vi "ASK Receiver.vi"() -> ()   [LabVIEW 2015]
uses:
  <vilib>/addons/Modulation/Analog/support/mod_Set Error Source.vi
  <vilib>/addons/Modulation/Digital/General/MT Generate ASK system parameters (M).vi
  <vilib>/addons/Modulation/Digital/Support/Common/Validators/mod_Generate Filter Coefficients Validate.vi
  <vilib>/addons/Modulation/Digital/General/subVIs/mod_Generate Filter Coefficients.vi
  <instrlib>/niUSRP/niUSRP Fetch Rx Data (CDB Cluster).vi
  <vilib>/addons/Modulation/niDMT.lvlib
panel:
  out "Waveform Graph":cluster{"t0":dbl, "dt":dbl, "Y":dbl[]}[](graph)
  out "XY Graph":T1(graph)
  out "output bit stream":i8[](array[numeric])
  out "Waveform Graph 2":i8[](graph)
  in  "synchronization parameters":T2 {"sync sequence" format="%.2f"}
  in  "pulse shaping filter (none)":T3(ring)
  in  "M-ASK (2)":i32=2
  in  "active antenna":string
  in  "number of samples":i64=1000
  out "coerced gain":dbl format="%#_6f"
  out "coerced carrier frequency":dbl=100000.0 format="%#_6p"
  out "coerced IQ rate":dbl=100000.0 format="%#_6p"
  in  "gain":dbl format="%#_6f"
  in  "carrier frequency":dbl=100000.0 format="%#_6p"
  in  "IQ rate":dbl=100000.0 format="%#_6p"
  in  "y":bool
  in  "device names":refnum<k15>
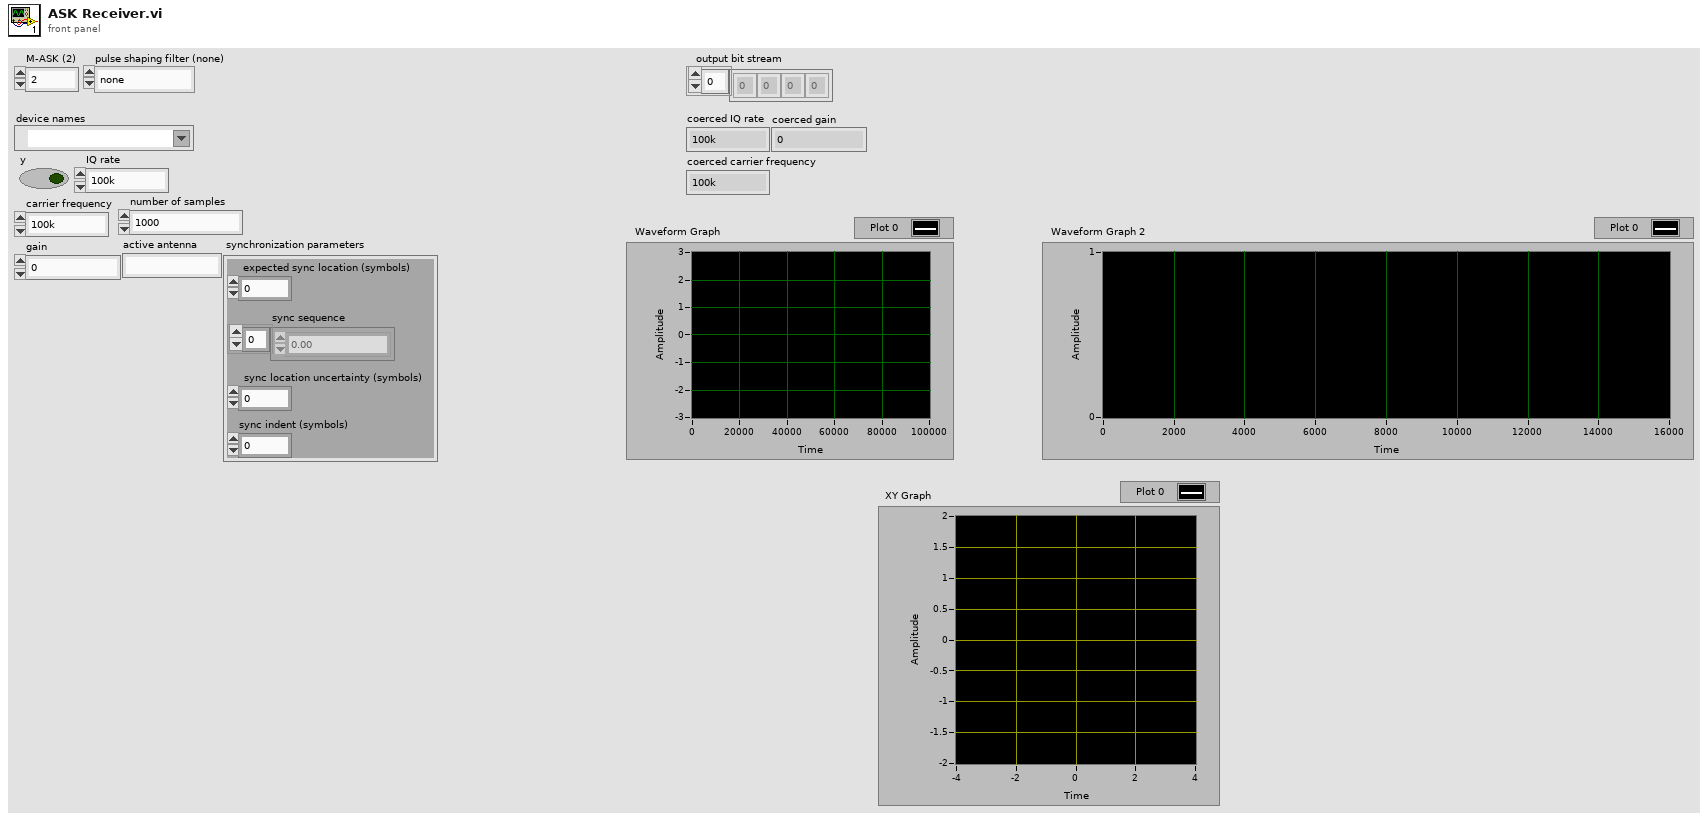
[diagram p1: front panel]
types:
  T1 = cluster{"constellation":dbl[], "oversampled data":dbl[]}[]
  T2 = cluster{"expected sync location (symbols)":i32, "sync sequence":cdb[], "sync location uncertainty (symbols)":i32, "sync indent (symbols)":i32}
  T3 = enum16{"none", "Raised Cosine", "Root Raised Cos", "Gaussian"}
  T4 = enum16{"FSK", "PSK", "QAM", "MSK", "PAM", "ASK", "CPM"}
  T5 = cluster{"samples per symbol (16)":i32, "symbol map":cdb[]}
  T6 = typedef "niAMT.lvlib/Complex Data Waveform.ctl" = cluster{"t0":dbl, "dt":dbl, "Y":cdb[]}
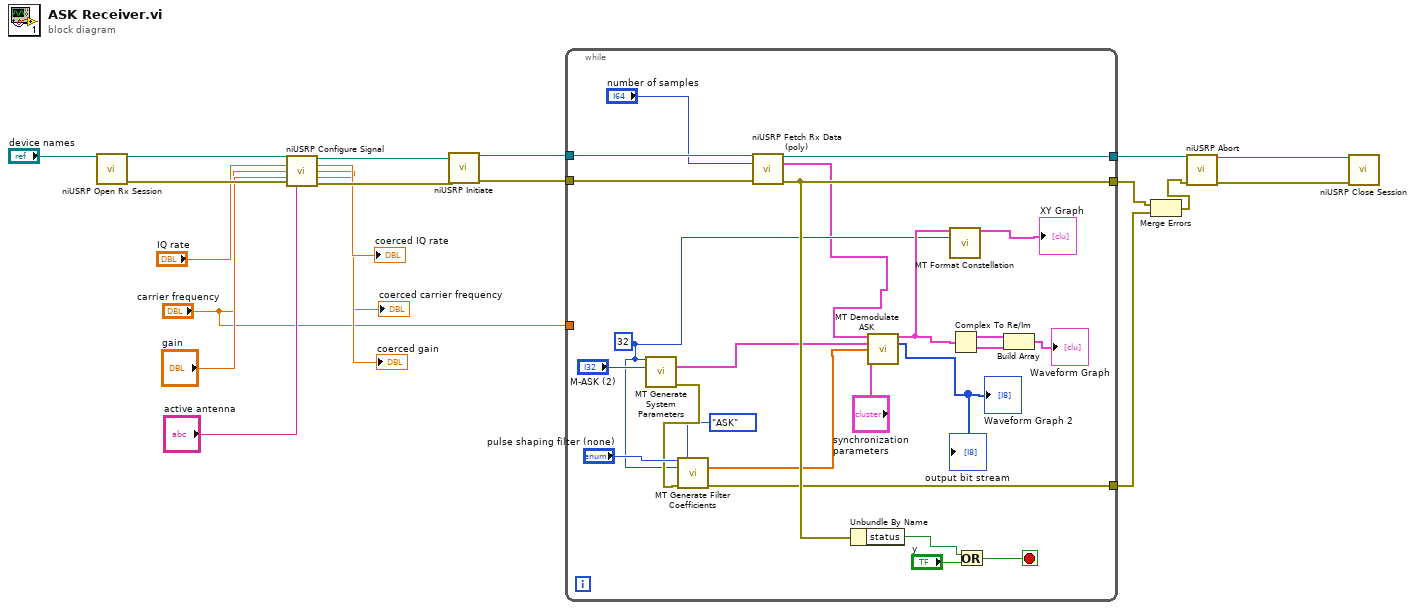
[diagram p0: block diagram]
diagram:
  n1 = call <instrlib>:"niUSRP Open Rx Session.vi"("device names"="device names") -> ("session handle out"=w19:refnum<k15>, "error out"=w17:errorcluster)  [unwired: 13 in]
  n2 = call <instrlib>:"niUSRP Configure Signal.vi"("session handle"=w19, "IQ rate"="IQ rate", "carrier frequency"="carrier frequency", "gain"="gain", "error in (no error)"=w17, "active antenna"="active antenna") -> ("session handle out"=w18:refnum<k15>, "coerced IQ rate"=→"coerced IQ rate":dbl, "coerced carrier frequency"=→"coerced carrier frequency":dbl, "coerced gain"=→"coerced gain":dbl, "error out"=w16:errorcluster)  [unwired: 5 in]
  n3 = call <instrlib>:"niUSRP Initiate.vi"("session handle"=w18, "error in (no error)"=w16) -> ("session handle out"=w15:refnum<k15>, "error out"=w12:errorcluster)  [unwired: 12 in]
  n4 = while {
    tunnel: w15 -> [w44]
    tunnel: [w43] -> w14
    tunnel: w12 -> [w42]
    tunnel: [w38] -> w3
    tunnel: "carrier frequency" -> [_]
    tunnel: [w29] -> w2
    stop <- w41 stop-if-true
    w23 = 32 ("samples per symbol (16)")
    n5 = call-poly <vilib>:"MT Generate System Parameters.vi"("samples per symbol (16)"=w23, "M-ASK (2)"="M-ASK (2)") -> ("ASK system parameters"=w34:T5, "error out"=w30:errorcluster)  [unwired: 11 in, 1 out]
    n6 = call <vilib>:"MT Generate Filter Coefficients.vi"("pulse shaping filter (none)"="pulse shaping filter (none)", "modulation type"=T4."ASK", "pulse shaping samples per symbol (16)"=w23, "error in (no error)"=w30) -> ("matched filter coefficients"=w32:dbl[], "error out"=w29:errorcluster)  [unwired: 9 in, 1 out]
    n7 = call-poly <instrlib>:"niUSRP Fetch Rx Data (poly).vi"("session handle"=w44, "number of samples"="number of samples", "error in (no error)"=w42) -> ("session handle out"=w43:refnum<k15>, "data"=w22:cluster{"t0":dbl, "dt":dbl, "Y":cdb[]}, "error out"=w38:errorcluster)  [unwired: 9 in, 1 out]
    n8 = Unbundle By Name(w38) -> ("status"=w39:bool)
    n9 = call <vilib>:"MT Demodulate ASK.vi"("input complex waveform"=w22, "ASK system parameters"=w34, "matched filter coefficients"=w32, "synchronization parameters"="synchronization parameters") -> ("recovered complex waveform"=w25:T6, "output bit stream"=→"Waveform Graph 2" →"output bit stream":i8[])  [unwired: 7 in, 3 out]
    n10 = call <vilib>:"MT Format Constellation.vi"("waveform"=w25, "samples per symbol"=w23) -> ("constellation graph"=→"XY Graph":T1)  [unwired: 12 in, 1 out]
    n11 = Complex To Re/Im(x + iy=w25) -> (x=w37:cluster{"t0":dbl, "dt":dbl, "Y":dbl[]}, y=w36:cluster{"t0":dbl, "dt":dbl, "Y":dbl[]})
    n12 = Or(x=w39, y="y") -> (x .or. y?=w41:bool)
    n13 = Build Array(w37, w36) -> (→"Waveform Graph":cluster{"t0":dbl, "dt":dbl, "Y":dbl[]}[])
  }
  n14 = Merge Errors(w3, w2) -> (w1:errorcluster)
  n15 = call <instrlib>:"niUSRP Abort.vi"("session handle"=w14, "error in (no error)"=w1) -> ("session handle out"=w13:refnum<k15>, "error out"=w11:errorcluster)  [unwired: 12 in]
  n16 = call <instrlib>:"niUSRP Close Session.vi"("session handle"=w13, "error in (no error)"=w11) -> ()  [unwired: 13 in, 1 out]
